vi "打码软件.vi"() -> ()   [LabVIEW 2017]
uses:
  <vilib>/Instr/_visa.llb/VISA Configure Serial Port (Instr).vi
  <vilib>/ptbypt/NI_PtbyPt.lvlib
panel:
  in  "监控":bool
  out "选项卡控件":enum32{"主选项卡", "监控"}(tab)
  in  "输入打标码后五位\n如：S0001":string
  in  "确定":bool
  out "当前打标码":string
  in  "手动打标":bool
  in  "停止":bool
  in  "退出":bool
  in  "PLC状态":bool
  out "串口通讯":bool
  out "PLC通讯":bool
  in  "返回":bool
  out "初始化回复":string
  out "打标模式回复":string
  out "初始条码":string
  out "打标V1写入回复":string
  out "打标V3写入回复":string
  out "开始打标写入回复":string
  out "停止打标回复":string
  in  "自动打标":bool
  out "错误输出 2":errorcluster caption="错误输出"
  out "元素":u32
  out "初始化文件回复":string
  # "SIC 打 标 软 件"
  # "自定义条码"
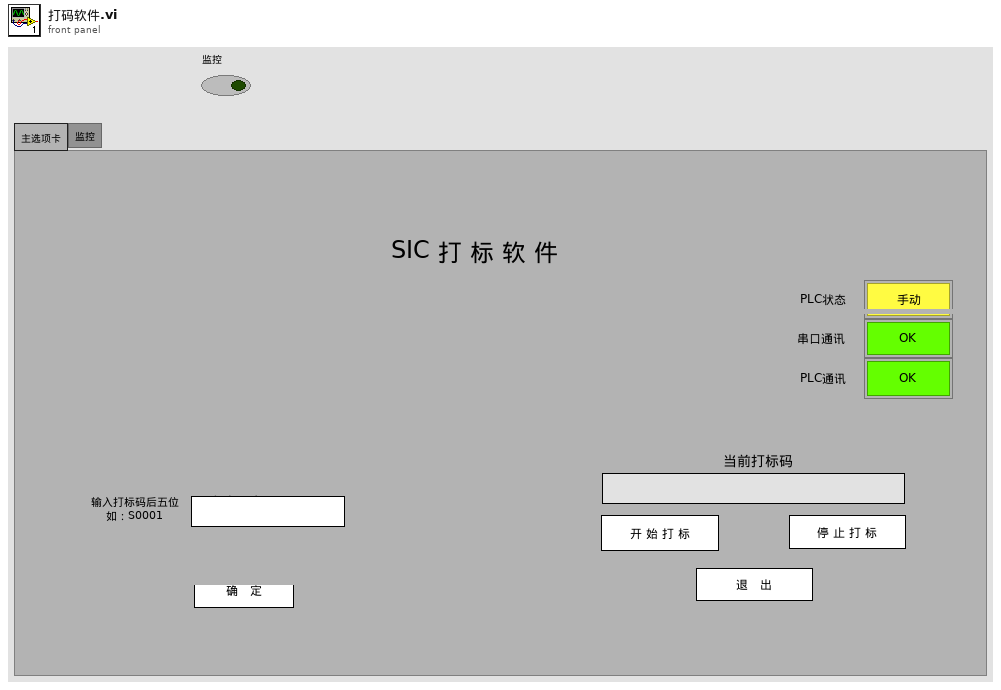
[diagram p1: front panel]
types:
  T1 = typedef "控件 1.ctl" = enum16{"通讯连接", "读PLC指令", "串口连接", "初始化", "打标模式", "事件", "错误", "退出"}
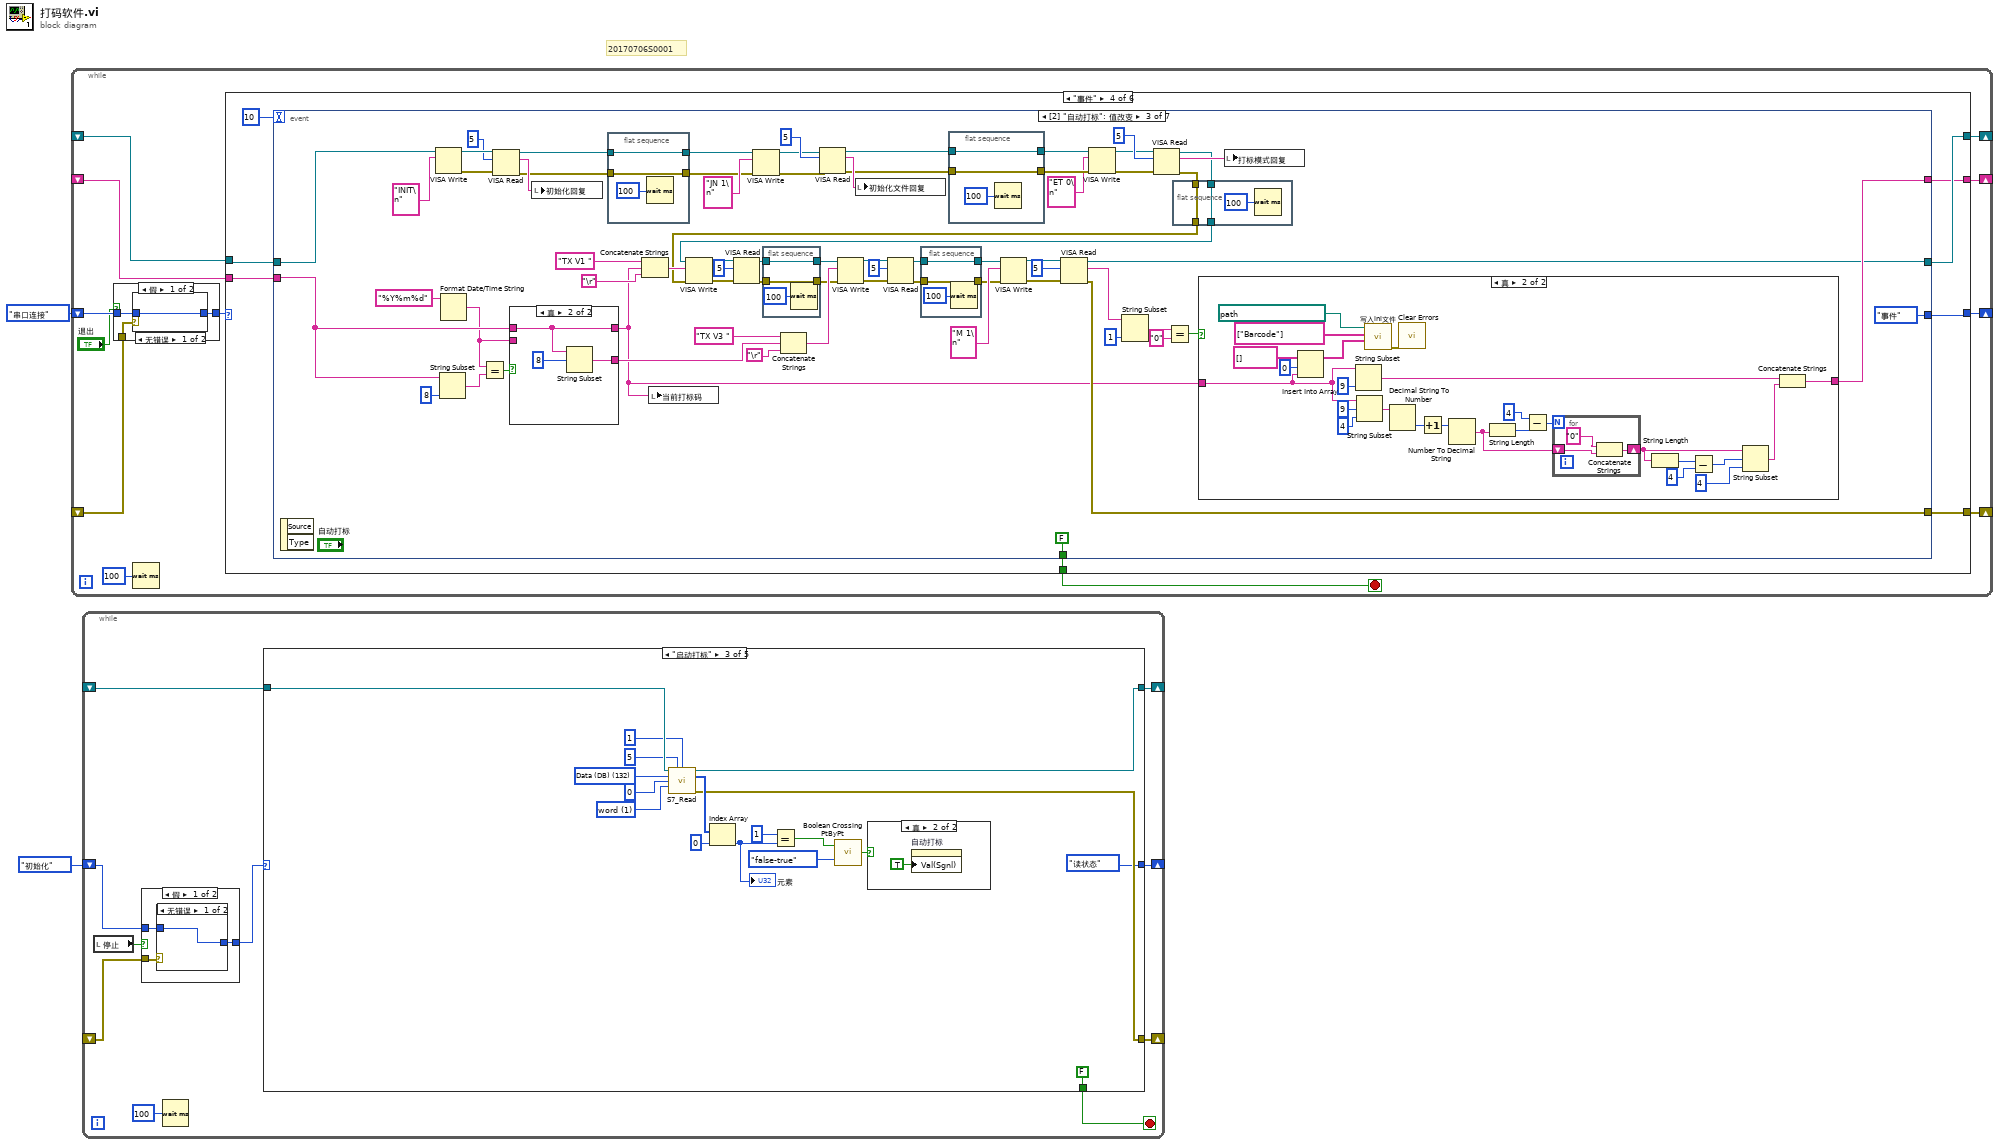
[diagram p0: block diagram]
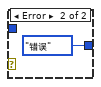
[diagram p2: hidden frame]
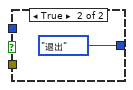
[diagram p3: hidden frame]
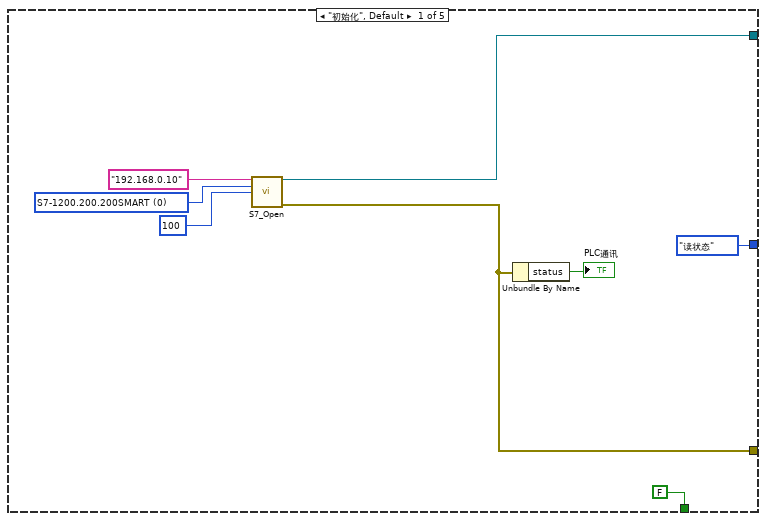
[diagram p4: hidden frame]
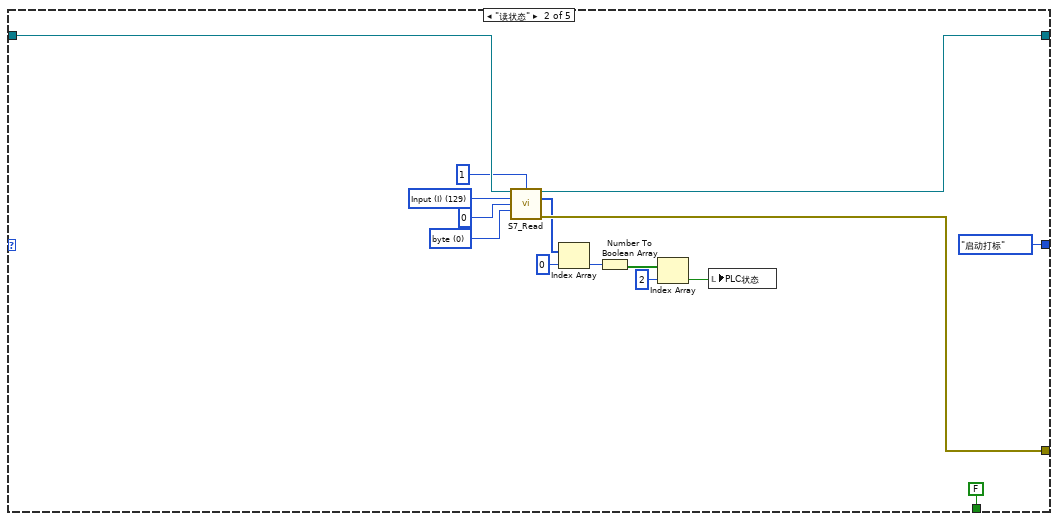
[diagram p5: hidden frame]
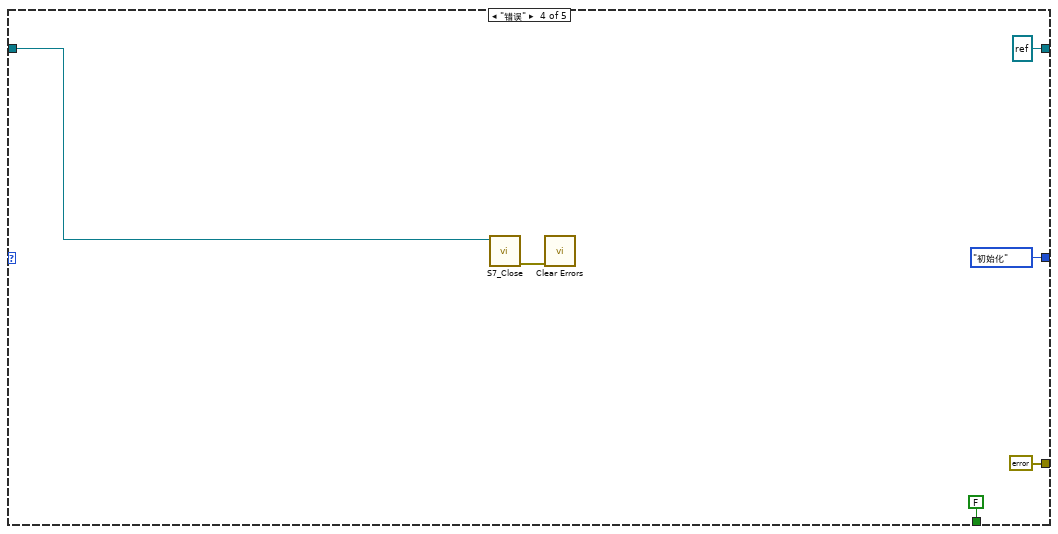
[diagram p7: hidden frame]
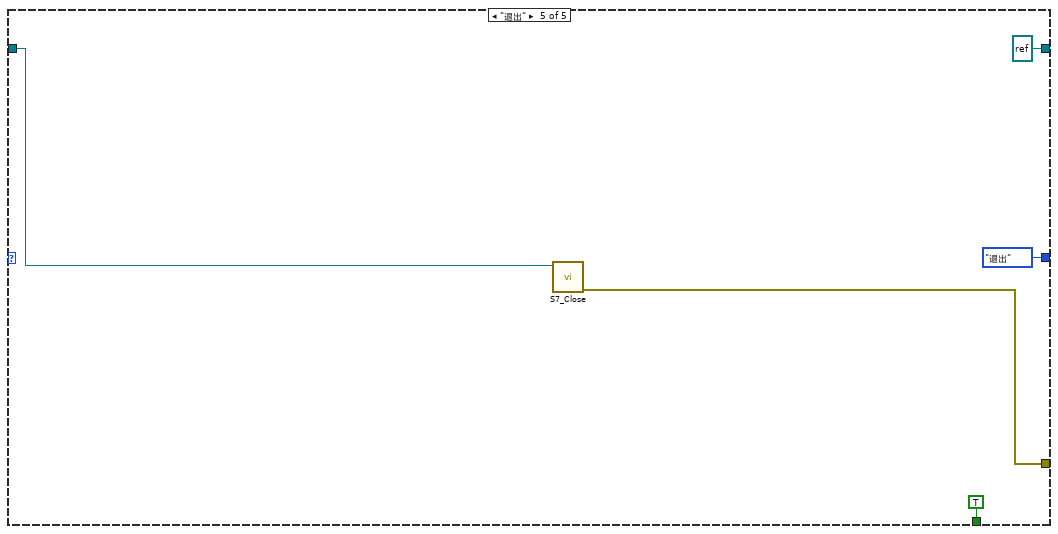
[diagram p8: hidden frame]
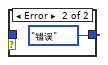
[diagram p9: hidden frame]
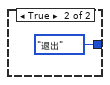
[diagram p10: hidden frame]
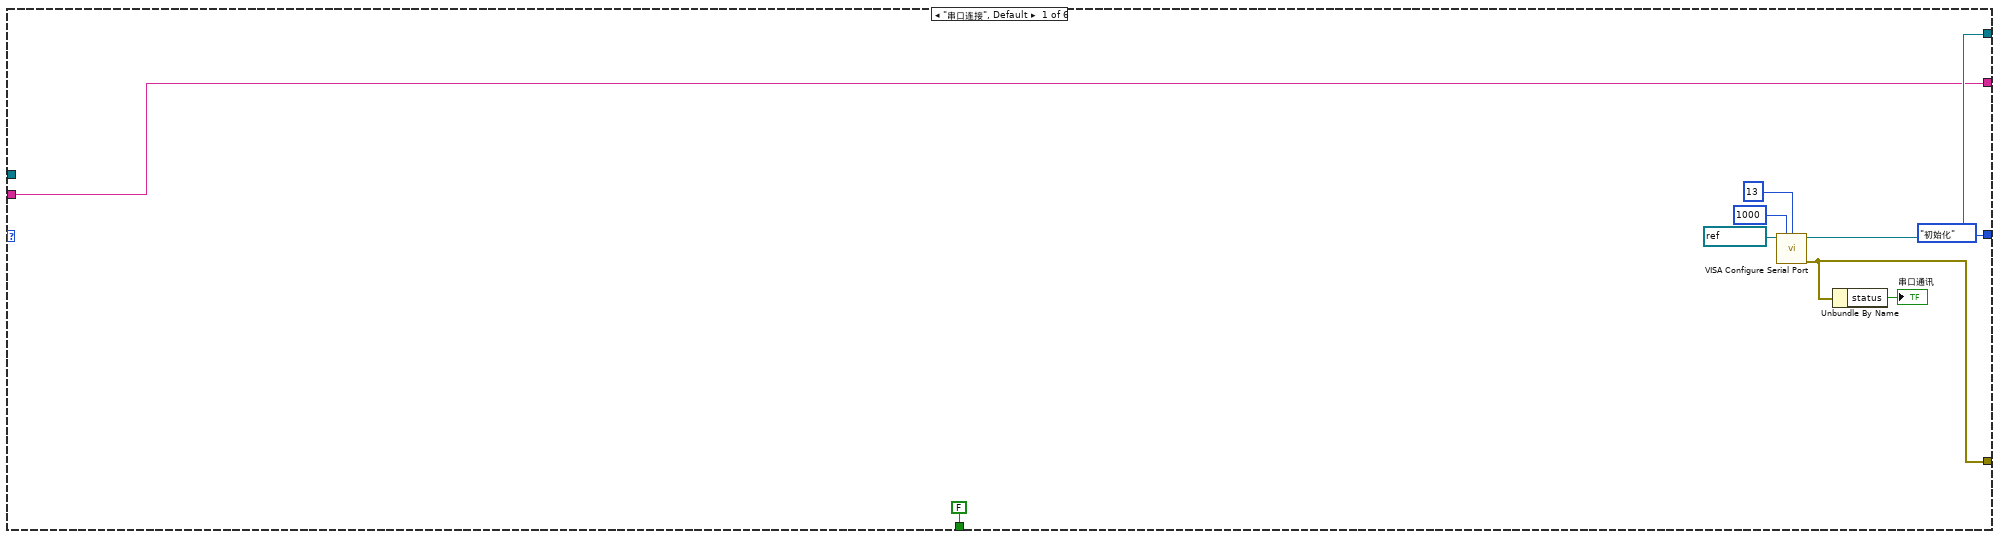
[diagram p11: hidden frame]
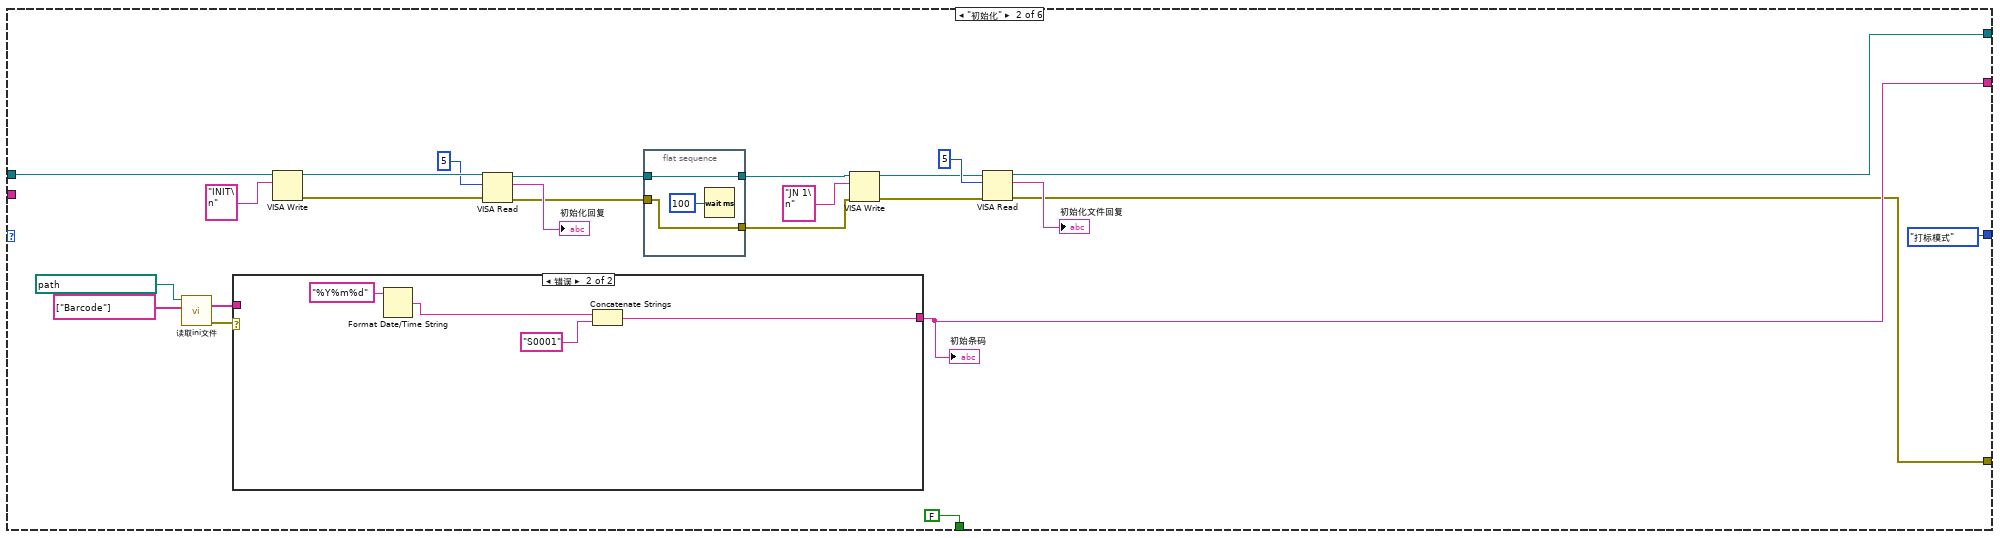
[diagram p12: hidden frame]
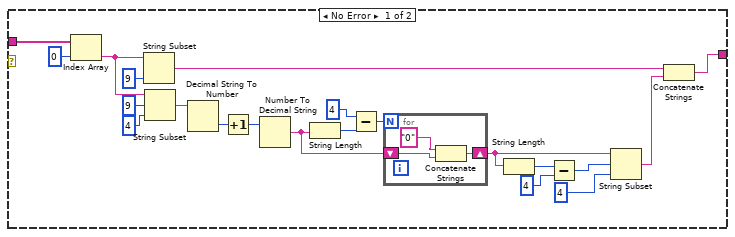
[diagram p13: hidden frame]
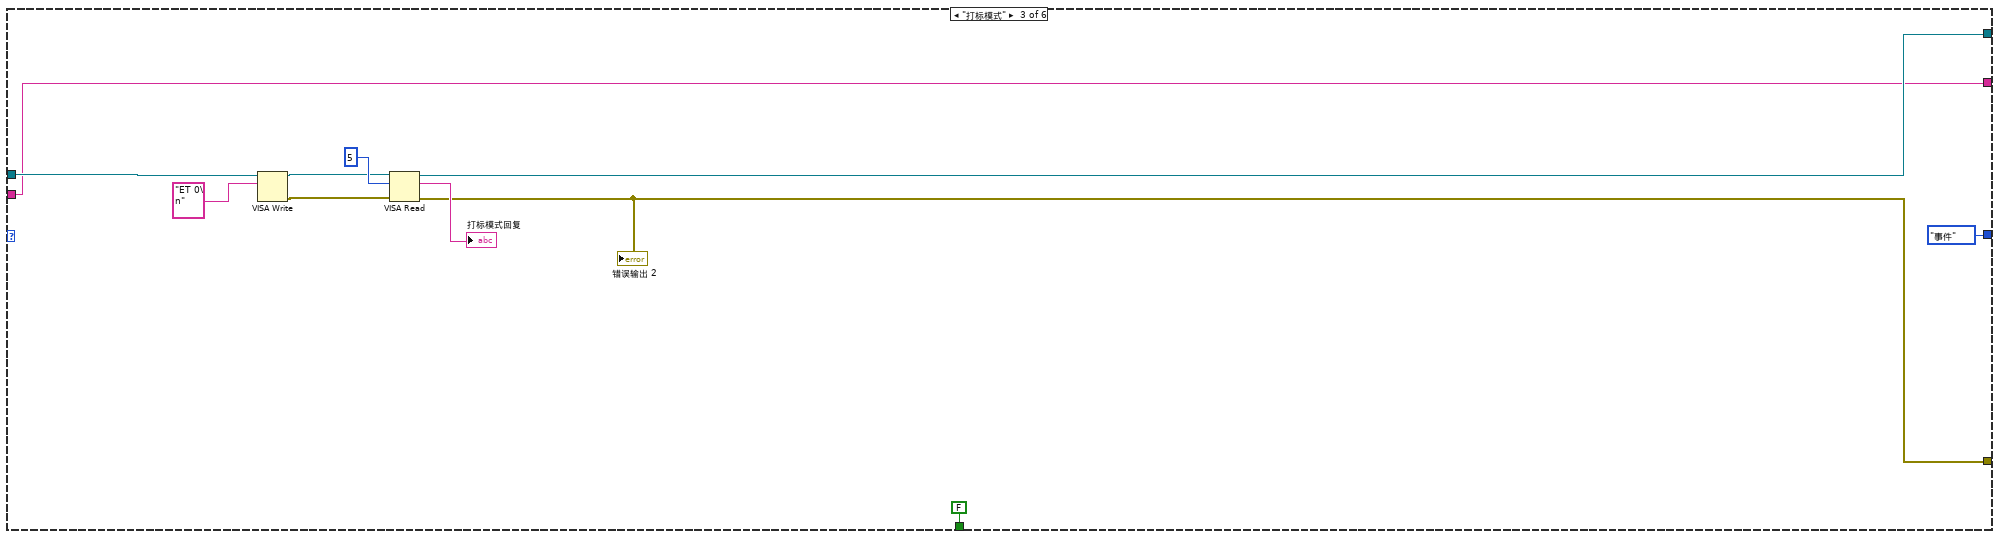
[diagram p14: hidden frame]
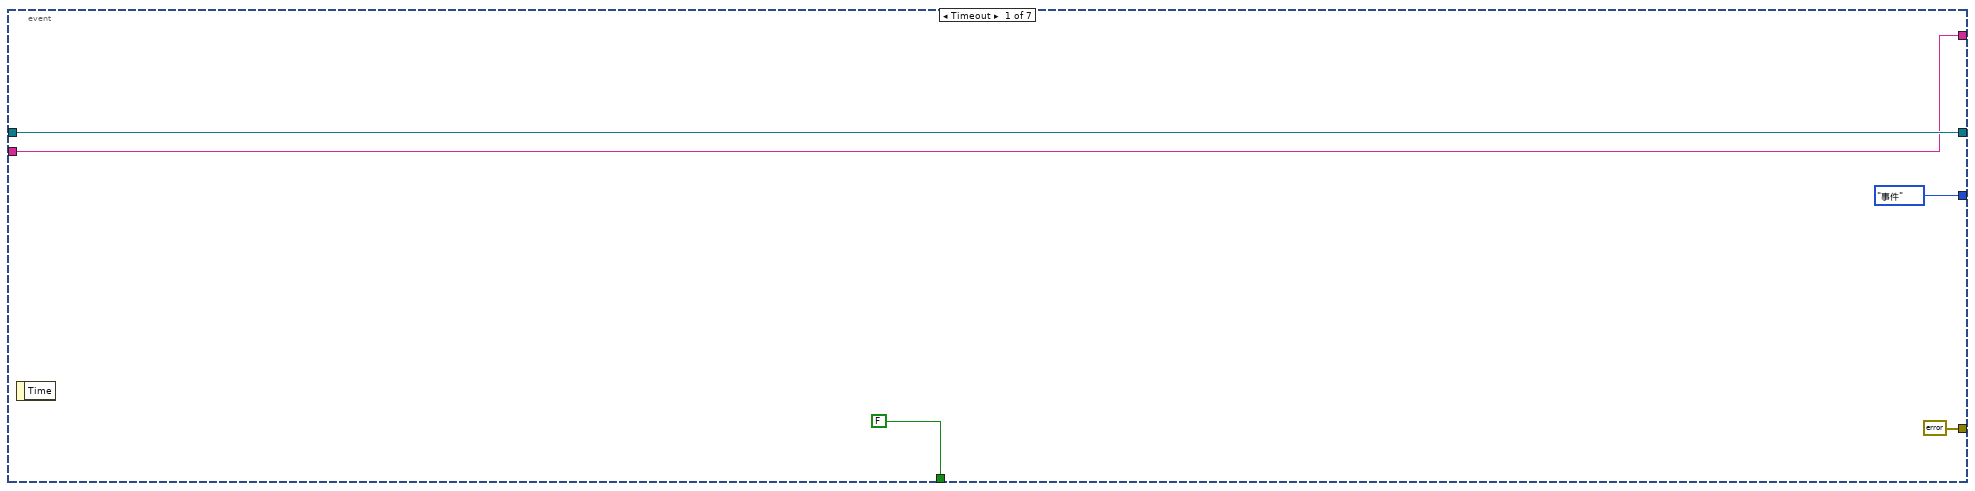
[diagram p15: hidden frame]
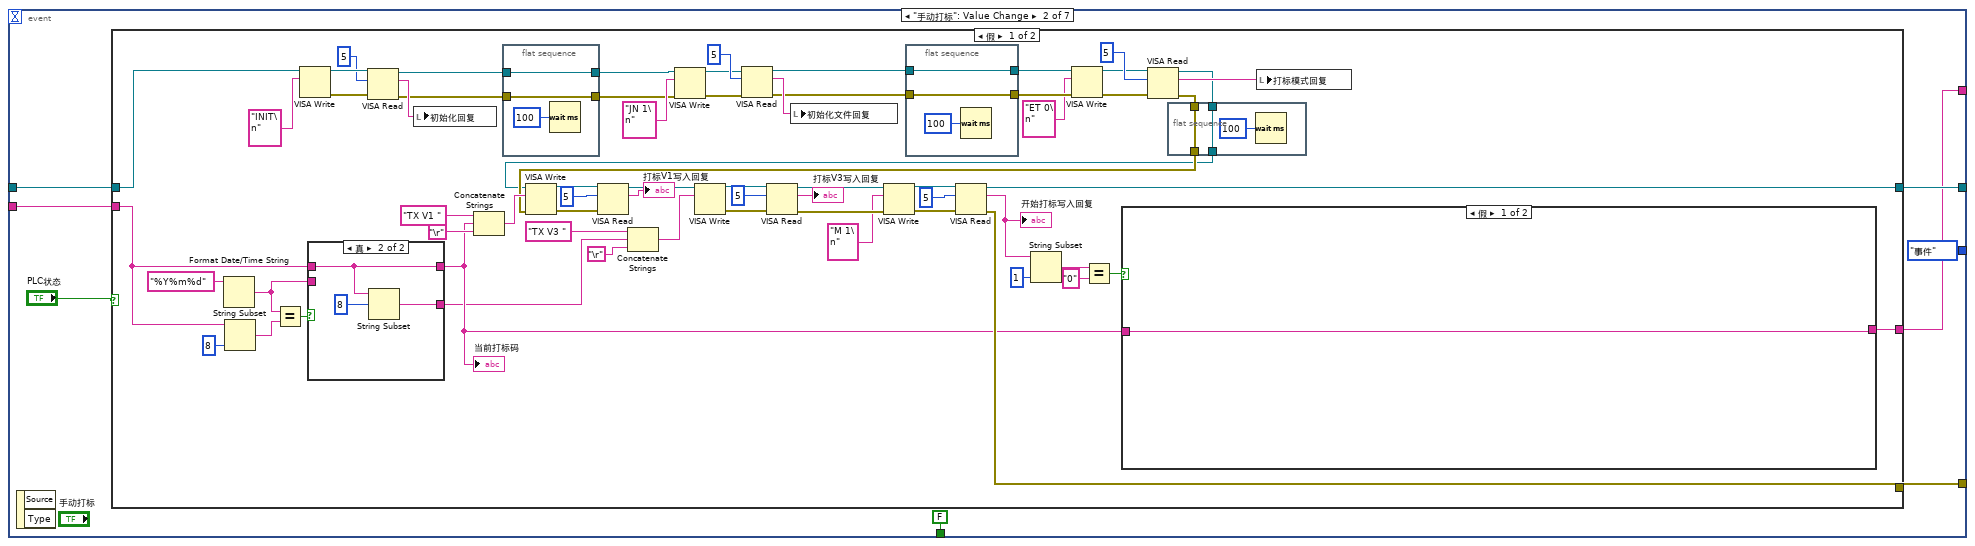
[diagram p16: hidden frame]
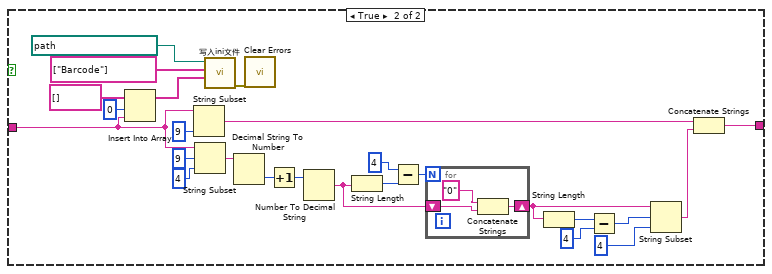
[diagram p17: hidden frame]
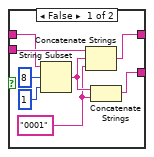
[diagram p18: hidden frame]
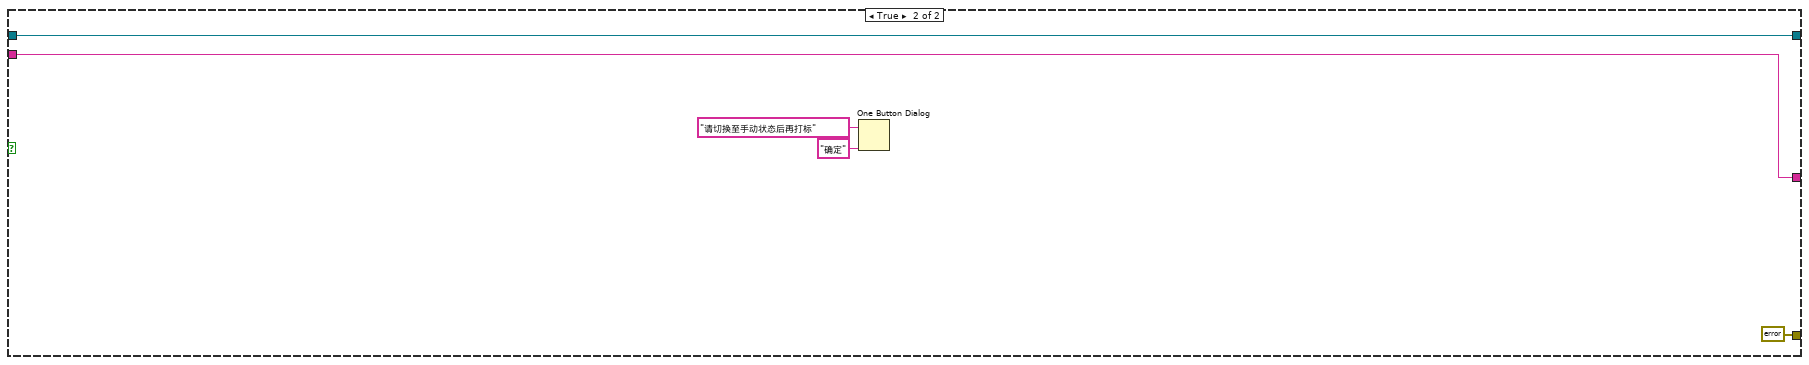
[diagram p19: hidden frame]
diagram:
  # "20170706S0001"
  n1 = while {
    shift-right: [w9] -> _
    shift-left: 控件_1."串口连接" -> [w14]
    shift-right: [w10] -> _
    shift-left: _ -> [w13]
    shift-right: [w11] -> _
    shift-left: _ -> [w8]
    shift-right: [w7] -> _
    shift-left: _ -> [w5]
    stop <- w6 stop-if-true
    n2 = case shown="假" "退出" {
      tunnel: w14 -> [w17 _]
      tunnel: w13 -> [w16 _]
      tunnel: [w15 控件_1."退出"] -> w12
      frame False {
        n3 = case shown="无错误" w16 {
          tunnel: w17 -> [w18 _]
          tunnel: [w18 控件_1."错误"] -> w15
          frame No Error {
          }
          frame Error {
          }
        }
      }
      frame True {
      }
    }
    n4 = Wait (ms)(milliseconds to wait=u32 100 ("等待时间（毫秒）")) -> ()  [unwired: 1 out]
    n5 = case shown="\"事件\"" w12 {
      tunnel: [w27 w31 w87 w99 refnum<visa-resource-name> refnum ("VISA resource name out") refnum<visa-resource-name> refnum ("VISA resource name out")] -> w11
      tunnel: [w24 w30 w88 w100 errorcluster {"status"=FALSE, "code"=0, "source"=""} ("error out") errorcluster {"status"=FALSE, "code"=0, "source"=""} ("error out")] -> w10
      tunnel: [控件_1."初始化" 控件_1."打标模式" 控件_1."事件" w97 控件_1."通讯连接" 控件_1."退出"] -> w9
      tunnel: w8 -> [_ w53 w94 w102 w397 w403]
      tunnel: [w22 w42 w85 w98 w395 ""] -> w7
      tunnel: [FALSE FALSE FALSE w96 FALSE TRUE] -> w6
      tunnel: w5 -> [w22 _ w85 w101 w395 _]
      frame "串口连接", Default {
        n6 = call-poly "VISA Configure Serial Port"("VISA resource name"=refnum<visa-resource-name> "COM1", "timeout (10sec)"=u32 1000, "termination char\n(0xA = '\\n' = LF)"=u8 13 ("termination char\n(0xA = '\\n' = LF)")) -> ("VISA resource name out"=w27:refnum<visa-resource-name>, "error out"=w24:errorcluster)  [unwired: 11 in]
        n7 = Unbundle By Name(w24) -> ("status"=→"串口通讯":bool)
      }
      frame "初始化" {
        n8 = call "读取ini文件.vi"("名称"=string[] ["Barcode"], "configuration file path"=path "D:/初始化文件/10.ini") -> ("error out"=w43:errorcluster, "值"=w44:string[])  [unwired: 8 in]
        n9 = case shown="错误" w43 {
          tunnel: w44 -> [w77 _]
          tunnel: [w57 w82] -> w42
          frame No Error {
            n10 = Index Array(array=w77, index=0 ("索引")) -> (element=w58:string)
            n11 = String Subset(string=w58, length (rest)=9 ("长度（剩余）")) -> (substring=w60:string)  [unwired: 1 in]
            n12 = String Subset(string=w58, offset (0)=9 ("偏移量(0)"), length (rest)=4 ("长度（剩余）")) -> (substring=w63:string)
            n13 = Decimal String To Number(string=w63) -> (number=w62:i32)  [unwired: 2 in, 1 out]
            n14 = Increment(x=w62) -> (x+1=w61:i32)
            n15 = Number To Decimal String(number=w61) -> (decimal integer string=w67:string)  [unwired: 1 in]
            n16 = String Length(string=w67) -> (length=w64:i32)
            n17 = Subtract(x=4, y=w64) -> (x-y=w66:i32)
            n18 = for {
              N: w66 -> [_]
              shift-right: [w80] -> w69
              shift-left: w67 -> [w79]
              n19 = Concatenate Strings("0" ("字符串"), w79) -> (w80:string)
            }
            n20 = String Length(string=w69) -> (length=w70:i32)
            n21 = Subtract(x=w70, y=4 ("x")) -> (x-y=w72:i32)
            n22 = String Subset(string=w69, offset (0)=w72, length (rest)=4 ("长度（剩余）")) -> (substring=w59:string)
            n23 = Concatenate Strings(w60, w59) -> (w57:string)
          }
          frame Error {
            n24 = Format Date/Time String(time format string (%c)="%Y%m%d" ("时间格式字符串(%c)")) -> (date/time string=w81:string)  [unwired: 2 in]
            n25 = Concatenate Strings(w81, "S0001" ("字符串")) -> (w82:string)
          }
        }
        "初始条码" <- w42
        n26 = VISA Write(VISA resource name=w53, write buffer="INIT\n" ("写入缓冲区")) -> (VISA resource name out=w50:refnum<visa-resource-name>, error out=w49:errorcluster)  [unwired: 1 in, 1 out]
        n27 = VISA Read(VISA resource name=w50, byte count=u32 5 ("字节总数"), error in (no error)=w49) -> (VISA resource name out=w37:refnum<visa-resource-name>, read buffer=→"初始化回复":string, error out=w35:errorcluster)  [unwired: 1 out]
        n28 = flat-sequence {
          tunnel: [w56] -> w36
          tunnel: w37 -> [w56]
          tunnel: w35 -> [w55]
          tunnel: [w55] -> w34
          frame #0 {
            n29 = Wait (ms)(milliseconds to wait=u32 100 ("等待时间（毫秒）")) -> ()  [unwired: 1 out]
          }
        }
        n30 = VISA Write(VISA resource name=w36, write buffer="JN 1\n" ("写入缓冲区"), error in (no error)=w34) -> (VISA resource name out=w33:refnum<visa-resource-name>, error out=w32:errorcluster)  [unwired: 1 out]
        n31 = VISA Read(VISA resource name=w33, byte count=u32 5 ("字节总数"), error in (no error)=w32) -> (VISA resource name out=w31:refnum<visa-resource-name>, read buffer=→"初始化文件回复":string, error out=w30:errorcluster)  [unwired: 1 out]
      }
      frame "打标模式" {
        n32 = VISA Write(VISA resource name=w94, write buffer="ET 0\n" ("写入缓冲区")) -> (VISA resource name out=w89:refnum<visa-resource-name>, error out=w90:errorcluster)  [unwired: 1 in, 1 out]
        n33 = VISA Read(VISA resource name=w89, byte count=u32 5 ("字节总数"), error in (no error)=w90) -> (VISA resource name out=w87:refnum<visa-resource-name>, read buffer=→"打标模式回复":string, error out=w88:errorcluster)  [unwired: 1 out]
        "错误输出 2" <- w88
      }
      frame "事件" {
        n34 = event shown="[2] \"自动打标\": 值改变" {
          selector: _ -> [_ _ _ _ _ _ _]
          dyn-events: _ -> [_ _ _ _ _ _ _]
          timeout: 10 -> [_ _ _ _ _ _ _]
          tunnel: w102 -> [w108 w116 w248 w367 w376 w384 w389]
          tunnel: w101 -> [w107 w115 w277 w363 _ w385 w388]
          tunnel: [errorcluster {"status"=FALSE, "code"=0, "source"=""} ("error out") w114 w276 w364 errorcluster {"status"=FALSE, "code"=0, "source"=""} ("error out") errorcluster {"status"=FALSE, "code"=0, "source"=""} ("error out") errorcluster {"status"=FALSE, "code"=0, "source"=""} ("error out")] -> w100
          tunnel: [w108 w113 w274 w365 w376 w384 w389] -> w99
          tunnel: [w107 w112 w275 w363 w377 w385 w388] -> w98
          tunnel: [控件_1."事件" 控件_1."事件" 控件_1."事件" 控件_1."事件" 控件_1."事件" 控件_1."事件" 控件_1."事件"] -> w97
          tunnel: [FALSE FALSE FALSE FALSE FALSE FALSE FALSE] -> w96
          event Timeout {
            n35 = event-data() -> ()  [unwired: 1 in, 1 out]
          }
          event "手动打标": Value Change {
            n36 = event-data() -> ()  [unwired: 1 in, 2 out]
            n37 = case shown="假" "PLC状态" {
              tunnel: w116 -> [w121 w234]
              tunnel: w115 -> [w173 w235]
              tunnel: [w150 errorcluster {"status"=FALSE, "code"=0, "source"=""} ("error out")] -> w114
              tunnel: [w149 w234] -> w113
              tunnel: [w147 w235] -> w112
              frame False {
                n38 = Format Date/Time String(time format string (%c)="%Y%m%d" ("时间格式字符串(%c)")) -> (date/time string=w146:string)  [unwired: 2 in]
                n39 = String Subset(string=w173, length (rest)=8 ("长度（剩余）")) -> (substring=w175:string)  [unwired: 1 in]
                n40 = Equal?(x=w146, y=w175) -> (x = y?=w174:bool)
                n41 = VISA Write(VISA resource name=w121, write buffer="INIT\n" ("写入缓冲区")) -> (VISA resource name out=w132:refnum<visa-resource-name>, error out=w131:errorcluster)  [unwired: 1 in, 1 out]
                n42 = case shown="真" w174 {
                  tunnel: w173 -> [w226 w230]
                  tunnel: [w223 w230] -> w148
                  tunnel: [w222 w228] -> w145
                  tunnel: w146 -> [w227 _]
                  frame False {
                    w220 = "0001"
                    n43 = String Subset(string=w226, offset (0)=8 ("偏移量(0)"), length (rest)=1 ("长度（剩余）")) -> (substring=w221:string)
                    n44 = Concatenate Strings(w227, w221, w220) -> (w223:string)
                    n45 = Concatenate Strings(w221, w220) -> (w222:string)
                  }
                  frame True {
                    n46 = String Subset(string=w230, offset (0)=8 ("偏移量(0)")) -> (substring=w228:string)  [unwired: 1 in]
                  }
                }
                "当前打标码" <- w148
                n47 = VISA Read(VISA resource name=w132, byte count=u32 5 ("字节总数"), error in (no error)=w131) -> (VISA resource name out=w127:refnum<visa-resource-name>, read buffer=w142:string, error out=w125:errorcluster)  [unwired: 1 out]
                n48 = local write "初始化回复"(w142) -> ()
                n49 = Concatenate Strings("TX V1 " ("写入缓冲区"), w148, "\r") -> (w170:string)
                n50 = flat-sequence {
                  tunnel: [w190] -> w126
                  tunnel: w127 -> [w190]
                  tunnel: w125 -> [w189]
                  tunnel: [w189] -> w124
                  frame #0 {
                    n51 = Wait (ms)(milliseconds to wait=u32 100 ("等待时间（毫秒）")) -> ()  [unwired: 1 out]
                  }
                }
                n52 = VISA Write(VISA resource name=w117, write buffer=w170, error in (no error)=w119) -> (VISA resource name out=w181:refnum<visa-resource-name>, error out=w180:errorcluster)  [unwired: 1 out]
                n53 = VISA Read(VISA resource name=w181, byte count=u32 5 ("字节总数"), error in (no error)=w180) -> (VISA resource name out=w163:refnum<visa-resource-name>, read buffer=→"打标V1写入回复":string)  [unwired: 2 out]
                n54 = Concatenate Strings("TX V3 " ("写入缓冲区"), w145, "\r") -> (w169:string)
                n55 = VISA Write(VISA resource name=w126, write buffer="JN 1\n" ("写入缓冲区"), error in (no error)=w124) -> (VISA resource name out=w123:refnum<visa-resource-name>, error out=w122:errorcluster)  [unwired: 1 out]
                n56 = VISA Write(VISA resource name=w163, write buffer=w169) -> (VISA resource name out=w164:refnum<visa-resource-name>, error out=w165:errorcluster)  [unwired: 1 in, 1 out]
                n57 = VISA Read(VISA resource name=w123, byte count=u32 5 ("字节总数"), error in (no error)=w122) -> (VISA resource name out=w138:refnum<visa-resource-name>, read buffer=w143:string, error out=w140:errorcluster)  [unwired: 1 out]
                n58 = VISA Read(VISA resource name=w164, byte count=u32 5 ("字节总数"), error in (no error)=w165) -> (VISA resource name out=w158:refnum<visa-resource-name>, read buffer=→"打标V3写入回复":string, error out=w157:errorcluster)  [unwired: 1 out]
                n59 = local write "初始化文件回复"(w143) -> ()
                n60 = VISA Write(VISA resource name=w158, write buffer="M 1\n" ("写入缓冲区"), error in (no error)=w157) -> (VISA resource name out=w161:refnum<visa-resource-name>, error out=w160:errorcluster)  [unwired: 1 out]
                n61 = flat-sequence {
                  tunnel: [w187] -> w139
                  tunnel: w138 -> [w187]
                  tunnel: [w186] -> w141
                  tunnel: w140 -> [w186]
                  frame #0 {
                    n62 = Wait (ms)(milliseconds to wait=u32 100 ("等待时间（毫秒）")) -> ()  [unwired: 1 out]
                  }
                }
                n63 = VISA Read(VISA resource name=w161, byte count=u32 5 ("字节总数"), error in (no error)=w160) -> (VISA resource name out=w149:refnum<visa-resource-name>, read buffer=w155:string, error out=w150:errorcluster)  [unwired: 1 out]
                "开始打标写入回复" <- w155
                n64 = String Subset(string=w155, length (rest)=1 ("长度（剩余）")) -> (substring=w153:string)  [unwired: 1 in]
                n65 = VISA Write(VISA resource name=w139, write buffer="ET 0\n" ("写入缓冲区"), error in (no error)=w141) -> (VISA resource name out=w134:refnum<visa-resource-name>, error out=w135:errorcluster)  [unwired: 1 out]
                n66 = Equal?(x=w153, y="0") -> (x = y?=w151:bool)
                n67 = case shown="假" w151 {
                  tunnel: w148 -> [w191 w193]
                  tunnel: [w191 w192] -> w147
                  frame False {
                  }
                  frame True {
                    n68 = Insert Into Array(array=string[] [] ("数组"), index=0 ("索引"), new element=w193) -> (w213:string[])
                    n69 = String Subset(string=w193, length (rest)=9 ("长度（剩余）")) -> (substring=w195:string)  [unwired: 1 in]
                    n70 = String Subset(string=w193, offset (0)=9 ("偏移量(0)"), length (rest)=4 ("长度（剩余）")) -> (substring=w198:string)
                    n71 = call "写入ini文件.vi"("值"=w213, "名称"=string[] ["Barcode"], "configuration file path"=path "D:/初始化文件/10.ini") -> ("error out"=w216:errorcluster)  [unwired: 8 in]
                    n72 = Decimal String To Number(string=w198) -> (number=w197:i32)  [unwired: 2 in, 1 out]
                    n73 = call <vilib>:"Clear Errors.vi"("error in (no error)"=w216) -> ()  [unwired: 5 in, 2 out]
                    n74 = Increment(x=w197) -> (x+1=w196:i32)
                    n75 = Number To Decimal String(number=w196) -> (decimal integer string=w202:string)  [unwired: 1 in]
                    n76 = String Length(string=w202) -> (length=w199:i32)
                    n77 = Subtract(x=4, y=w199) -> (x-y=w201:i32)
                    n78 = for {
                      N: w201 -> [_]
                      shift-right: [w219] -> w204
                      shift-left: w202 -> [w218]
                      n79 = Concatenate Strings("0" ("字符串"), w218) -> (w219:string)
                    }
                    n80 = String Length(string=w204) -> (length=w205:i32)
                    n81 = Subtract(x=w205, y=4 ("x")) -> (x-y=w207:i32)
                    n82 = String Subset(string=w204, offset (0)=w207, length (rest)=4 ("长度（剩余）")) -> (substring=w194:string)
                    n83 = Concatenate Strings(w195, w194) -> (w192:string)
                  }
                }
                n84 = VISA Read(VISA resource name=w134, byte count=u32 5 ("字节总数"), error in (no error)=w135) -> (VISA resource name out=w118:refnum<visa-resource-name>, read buffer=w144:string, error out=w120:errorcluster)  [unwired: 1 out]
                n85 = flat-sequence {
                  tunnel: w118 -> [w184]
                  tunnel: [w184] -> w117
                  tunnel: w120 -> [w183]
                  tunnel: [w183] -> w119
                  frame #0 {
                    n86 = Wait (ms)(milliseconds to wait=u32 100 ("等待时间（毫秒）")) -> ()  [unwired: 1 out]
                  }
                }
                n87 = local write "打标模式回复"(w144) -> ()
              }
              frame True {
                n88 = One Button Dialog(message="请切换至手动状态后再打标" ("消息"), button name ("OK")="确定" ("按钮名称（“确定”）")) -> ()  [unwired: 1 out]
              }
            }
          }
          event "自动打标": Value Change {
            n89 = event-data() -> ()  [unwired: 1 in, 2 out]
            n90 = VISA Write(VISA resource name=w248, write buffer="INIT\n" ("写入缓冲区")) -> (VISA resource name out=w259:refnum<visa-resource-name>, error out=w258:errorcluster)  [unwired: 1 in, 1 out]
            n91 = String Subset(string=w277, length (rest)=8 ("长度（剩余）")) -> (substring=w298:string)  [unwired: 1 in]
            n92 = Format Date/Time String(time format string (%c)="%Y%m%d" ("时间格式字符串(%c)")) -> (date/time string=w272:string)  [unwired: 2 in]
            n93 = Equal?(x=w272, y=w298) -> (x = y?=w297:bool)
            n94 = VISA Read(VISA resource name=w259, byte count=u32 5 ("字节总数"), error in (no error)=w258) -> (VISA resource name out=w254:refnum<visa-resource-name>, read buffer=w269:string, error out=w252:errorcluster)  [unwired: 1 out]
            n95 = case shown="真" w297 {
              tunnel: w277 -> [w356 w360]
              tunnel: [w353 w360] -> w273
              tunnel: [w352 w358] -> w287
              tunnel: w272 -> [w357 _]
              frame False {
                w350 = "0001"
                n96 = String Subset(string=w356, offset (0)=8 ("偏移量(0)"), length (rest)=1 ("长度（剩余）")) -> (substring=w351:string)
                n97 = Concatenate Strings(w357, w351, w350) -> (w353:string)
                n98 = Concatenate Strings(w351, w350) -> (w352:string)
              }
              frame True {
                n99 = String Subset(string=w360, offset (0)=8 ("偏移量(0)")) -> (substring=w358:string)  [unwired: 1 in]
              }
            }
            n100 = local write "初始化回复"(w269) -> ()
            n101 = flat-sequence {
              tunnel: [w320] -> w253
              tunnel: w254 -> [w320]
              tunnel: w252 -> [w319]
              tunnel: [w319] -> w251
              frame #0 {
                n102 = Wait (ms)(milliseconds to wait=u32 100 ("等待时间（毫秒）")) -> ()  [unwired: 1 out]
              }
            }
            n103 = Concatenate Strings("TX V1 " ("写入缓冲区"), w273, "\r") -> (w294:string)
            n104 = local write "当前打标码"(w273) -> ()
            n105 = VISA Write(VISA resource name=w246, write buffer=w294, error in (no error)=w244) -> (VISA resource name out=w303:refnum<visa-resource-name>, error out=w302:errorcluster)  [unwired: 1 out]
            n106 = VISA Read(VISA resource name=w303, byte count=u32 5 ("字节总数"), error in (no error)=w302) -> (VISA resource name out=w243:refnum<visa-resource-name>, error out=w241:errorcluster)  [unwired: 2 out]
            n107 = VISA Write(VISA resource name=w253, write buffer="JN 1\n" ("写入缓冲区"), error in (no error)=w251) -> (VISA resource name out=w250:refnum<visa-resource-name>, error out=w249:errorcluster)  [unwired: 1 out]
            n108 = flat-sequence {
              tunnel: w243 -> [w311]
              tunnel: [w311] -> w242
              tunnel: w241 -> [w310]
              tunnel: [w310] -> w240
              frame #0 {
                n109 = Wait (ms)(milliseconds to wait=u32 100 ("等待时间（毫秒）")) -> ()  [unwired: 1 out]
              }
            }
            n110 = Concatenate Strings("TX V3 " ("写入缓冲区"), w287, "\r") -> (w293:string)
            n111 = VISA Read(VISA resource name=w250, byte count=u32 5 ("字节总数"), error in (no error)=w249) -> (VISA resource name out=w265:refnum<visa-resource-name>, read buffer=w270:string, error out=w267:errorcluster)  [unwired: 1 out]
            n112 = VISA Write(VISA resource name=w242, write buffer=w293, error in (no error)=w240) -> (VISA resource name out=w288:refnum<visa-resource-name>, error out=w289:errorcluster)  [unwired: 1 out]
            n113 = local write "初始化文件回复"(w270) -> ()
            n114 = VISA Read(VISA resource name=w288, byte count=u32 5 ("字节总数"), error in (no error)=w289) -> (VISA resource name out=w238:refnum<visa-resource-name>, error out=w239:errorcluster)  [unwired: 2 out]
            n115 = flat-sequence {
              tunnel: w238 -> [w308]
              tunnel: [w308] -> w237
              tunnel: w239 -> [w307]
              tunnel: [w307] -> w236
              frame #0 {
                n116 = Wait (ms)(milliseconds to wait=u32 100 ("等待时间（毫秒）")) -> ()  [unwired: 1 out]
              }
            }
            n117 = flat-sequence {
              tunnel: [w317] -> w266
              tunnel: w265 -> [w317]
              tunnel: [w316] -> w268
              tunnel: w267 -> [w316]
              frame #0 {
                n118 = Wait (ms)(milliseconds to wait=u32 100 ("等待时间（毫秒）")) -> ()  [unwired: 1 out]
              }
            }
            n119 = VISA Write(VISA resource name=w237, write buffer="M 1\n" ("写入缓冲区"), error in (no error)=w236) -> (VISA resource name out=w286:refnum<visa-resource-name>, error out=w285:errorcluster)  [unwired: 1 out]
            n120 = VISA Read(VISA resource name=w286, byte count=u32 5 ("字节总数"), error in (no error)=w285) -> (VISA resource name out=w274:refnum<visa-resource-name>, read buffer=w282:string, error out=w276:errorcluster)  [unwired: 1 out]
            n121 = VISA Write(VISA resource name=w266, write buffer="ET 0\n" ("写入缓冲区"), error in (no error)=w268) -> (VISA resource name out=w261:refnum<visa-resource-name>, error out=w262:errorcluster)  [unwired: 1 out]
            n122 = String Subset(string=w282, length (rest)=1 ("长度（剩余）")) -> (substring=w280:string)  [unwired: 1 in]
            n123 = VISA Read(VISA resource name=w261, byte count=u32 5 ("字节总数"), error in (no error)=w262) -> (VISA resource name out=w247:refnum<visa-resource-name>, read buffer=w271:string, error out=w245:errorcluster)  [unwired: 1 out]
            n124 = Equal?(x=w280, y="0") -> (x = y?=w278:bool)
            n125 = flat-sequence {
              tunnel: w247 -> [w314]
              tunnel: [w314] -> w246
              tunnel: w245 -> [w313]
              tunnel: [w313] -> w244
              frame #0 {
                n126 = Wait (ms)(milliseconds to wait=u32 100 ("等待时间（毫秒）")) -> ()  [unwired: 1 out]
              }
            }
            n127 = case shown="真" w278 {
              tunnel: w273 -> [w321 w323]
              tunnel: [w321 w322] -> w275
              frame False {
              }
              frame True {
                n128 = Insert Into Array(array=string[] [] ("数组"), index=0 ("索引"), new element=w323) -> (w343:string[])
                n129 = String Subset(string=w323, length (rest)=9 ("长度（剩余）")) -> (substring=w325:string)  [unwired: 1 in]
                n130 = String Subset(string=w323, offset (0)=9 ("偏移量(0)"), length (rest)=4 ("长度（剩余）")) -> (substring=w328:string)
                n131 = call "写入ini文件.vi"("值"=w343, "名称"=string[] ["Barcode"], "configuration file path"=path "D:/初始化文件/10.ini") -> ("error out"=w346:errorcluster)  [unwired: 8 in]
                n132 = Decimal String To Number(string=w328) -> (number=w327:i32)  [unwired: 2 in, 1 out]
                n133 = call <vilib>:"Clear Errors.vi"("error in (no error)"=w346) -> ()  [unwired: 5 in, 2 out]
                n134 = Increment(x=w327) -> (x+1=w326:i32)
                n135 = Number To Decimal String(number=w326) -> (decimal integer string=w332:string)  [unwired: 1 in]
                n136 = String Length(string=w332) -> (length=w329:i32)
                n137 = Subtract(x=4, y=w329) -> (x-y=w331:i32)
                n138 = for {
                  N: w331 -> [_]
                  shift-right: [w349] -> w334
                  shift-left: w332 -> [w348]
                  n139 = Concatenate Strings("0" ("字符串"), w348) -> (w349:string)
                }
                n140 = String Length(string=w334) -> (length=w335:i32)
                n141 = Subtract(x=w335, y=4 ("x")) -> (x-y=w337:i32)
                n142 = String Subset(string=w334, offset (0)=w337, length (rest)=4 ("长度（剩余）")) -> (substring=w324:string)
                n143 = Concatenate Strings(w325, w324) -> (w322:string)
              }
            }
            n144 = local write "打标模式回复"(w271) -> ()
          }
          event "停止": Value Change {
            n145 = event-data() -> ()  [unwired: 1 in, 2 out]
            n146 = VISA Write(VISA resource name=w367, write buffer="M 0\n" ("写入缓冲区")) -> (VISA resource name out=w371:refnum<visa-resource-name>, error out=w370:errorcluster)  [unwired: 1 in, 1 out]
            n147 = VISA Read(VISA resource name=w371, byte count=u32 5 ("字节总数"), error in (no error)=w370) -> (VISA resource name out=w365:refnum<visa-resource-name>, read buffer=→"停止打标回复":string, error out=w364:errorcluster)  [unwired: 1 out]
          }
          event "确定": Value Change {
            n148 = event-data() -> ()  [unwired: 1 in, 2 out]
            n149 = Format Date/Time String(time format string (%c)="%Y%m%d" ("时间格式字符串(%c)")) -> (date/time string=w372:string)  [unwired: 2 in]
            n150 = Concatenate Strings(w372, "输入打标码后五位\n如：S0001") -> (w377:string)
          }
          event "监控": Value Change {
            n151 = event-data() -> ()  [unwired: 1 in, 4 out]
            "选项卡控件" <- enum32{"主选项卡", "监控"}."监控" ("选项卡控件")
          }
          event "返回": Value Change {
            n152 = event-data() -> ()  [unwired: 1 in, 4 out]
            n153 = local write "选项卡控件"(enum32{"主选项卡", "监控"}."主选项卡" ("选项卡控件")) -> ()
          }
        }
      }
      frame "错误" {
        n154 = VISA Close(VISA resource name=w397) -> ()  [unwired: 1 in, 1 out]
      }
      frame "退出" {
        n155 = VISA Close(VISA resource name=w403) -> (error out=w404:errorcluster)  [unwired: 1 in]
        n156 = call <vilib>:"Clear Errors.vi"("error in (no error)"=w404) -> ()  [unwired: 5 in, 2 out]
        n157 = control-ref of="本VI"() -> (w405:refnum<vi>)
        n158 = invoke class="VI" method="FP.Close"(reference=w405) -> ()  [unwired: 2 in, 3 out]
      }
    }
  }
  n159 = while {
    shift-right: [w414] -> _
    shift-left: _ -> [w411]
    shift-right: [w413] -> _
    shift-left: _ -> [w409]
    shift-right: [w412] -> _
    shift-left: enum16{"初始化", "读状态", "启动打标", "错误", "退出"}."初始化" -> [w408]
    stop <- w410 stop-if-true
    n160 = local read "停止"() -> (w415:bool)
    n161 = case shown="假" w415 {
      tunnel: [w417 enum16{"初始化", "读状态", "启动打标", "错误", "退出"}."退出"] -> w407
      tunnel: w409 -> [w418 _]
      tunnel: w408 -> [w416 _]
      frame False {
        n162 = case shown="无错误" w418 {
          tunnel: [w419 enum16{"初始化", "读状态", "启动打标", "错误", "退出"}."错误"] -> w417
          tunnel: w416 -> [w419 _]
          frame No Error {
          }
          frame Error {
          }
        }
      }
      frame True {
      }
    }
    n163 = Wait (ms)(milliseconds to wait=u32 100 ("等待时间（毫秒）")) -> ()  [unwired: 1 out]
    n164 = case shown="\"启动打标\"" w407 {
      tunnel: [w425 w439 w455 refnum<k5> refnum ("TCP") refnum<k5> refnum ("TCP")] -> w414
      tunnel: [w424 w440 w454 errorcluster {"status"=FALSE, "code"=0, "source"=""} ("error out") w472] -> w413
      tunnel: [enum16{"初始化", "读状态", "启动打标", "错误", "退出"}."读状态" enum16{"初始化", "读状态", "启动打标", "错误", "退出"}."启动打标" enum16{"初始化", "读状态", "启动打标", "错误", "退出"}."读状态" enum16{"初始化", "读状态", "启动打标", "错误", "退出"}."初始化" enum16{"初始化", "读状态", "启动打标", "错误", "退出"}."退出"] -> w412
      tunnel: w411 -> [_ w444 w456 w468 w473]
      tunnel: [FALSE FALSE FALSE FALSE TRUE] -> w410
      frame "初始化", Default {
        w428 = u8 0 items=["S7-1200.200.200SMART"=0, "S7-300"=2, "S7-400"=3] ("PLC 系列")
        n165 = call "S7_Open.vi"("IP 地址"="192.168.0.10", "PLC 系列"=w428, "超时（MS）"=100) -> ("TCP"=w425:refnum<k5>, "error out"=w424:errorcluster)  [unwired: 10 in, 1 out]
        n166 = Unbundle By Name(w424) -> ("status"=→"PLC通讯":bool)
      }
      frame "读状态" {
        w441 = u16 0 items=["byte", "word", "Dword"] ("数据类型")
        w443 = u8 129 items=["I/O (P)"=128, "Input (I)"=129, "Output (Q)"=130, "Bit Memory (M)"=131, "Data (DB)"=132, "Instance Data (DI)"=133, "Local Data (L)"=134, "Predecessor Local Data (VL)"=135] ("寄存器类型")
        n167 = call "S7_Read.vi"("TCP"=w444, "读取长度"=u16 1, "寄存器类型"=w443, "起始地址"=u32 0, "数据类型"=w441) -> ("TCP"=w439:refnum<k5>, "数据"=w438:u32[], "error out"=w440:errorcluster)  [unwired: 7 in, 1 out]
        n168 = Index Array(array=w438, index=0 ("索引")) -> (element=w433:u32)
        n169 = Number To Boolean Array(number=w433) -> (Boolean array=w432:bool[])
        n170 = Index Array(array=w432, index=2 ("索引")) -> (element=w430:bool)
        n171 = local write "PLC状态"(w430) -> ()
      }
      frame "启动打标" {
        w459 = u16 1 items=["byte", "word", "Dword"] ("数据类型")
        w461 = u8 132 items=["I/O (P)"=128, "Input (I)"=129, "Output (Q)"=130, "Bit Memory (M)"=131, "Data (DB)"=132, "Instance Data (DI)"=133, "Local Data (L)"=134, "Predecessor Local Data (VL)"=135] ("寄存器类型")
        n172 = call "S7_Read.vi"("TCP"=w456, "DB #"=u16 5, "读取长度"=u16 1, "寄存器类型"=w461, "起始地址"=u32 0, "数据类型"=w459) -> ("TCP"=w455:refnum<k5>, "数据"=w458:u32[], "error out"=w454:errorcluster)  [unwired: 6 in, 1 out]
        n173 = Index Array(array=w458, index=0 ("索引")) -> (element=w447:u32)
        "元素" <- w447
        n174 = Equal?(x=u32 1, y=w447) -> (x = y?=w445:bool)
        n175 = call <vilib>:"Boolean Crossing PtByPt.vi"("direction"=enum16{"either", "false-true", "true-false"}."false-true", "input"=w445) -> ("crossing"=w450:bool)  [unwired: 1 in]
        n176 = case shown="真" w450 {
          frame False {
          }
          frame True {
            n177 = property on="自动打标" class="Bool (严格)"("Val(Sgnl)"=TRUE ("值(信号)")) -> ()  [unwired: 2 in, 2 out]
          }
        }
      }
      frame "错误" {
        n178 = call "S7_Close.vi"("TCP Connection Ref"=w468) -> ("error out"=w464:errorcluster)  [unwired: 10 in]
        n179 = call <vilib>:"Clear Errors.vi"("error in (no error)"=w464) -> ()  [unwired: 5 in, 2 out]
      }
      frame "退出" {
        n180 = call "S7_Close.vi"("TCP Connection Ref"=w473) -> ("error out"=w472:errorcluster)  [unwired: 10 in]
      }
    }
  }
